vi "check should fail.vi"() -> ()   [LabVIEW 2017]
uses:
  Source/JSON Support for LabVIEW.lvlib
panel:
  out "Array":T1(array[cluster])
  # "Read as"
  # "Parsed As"
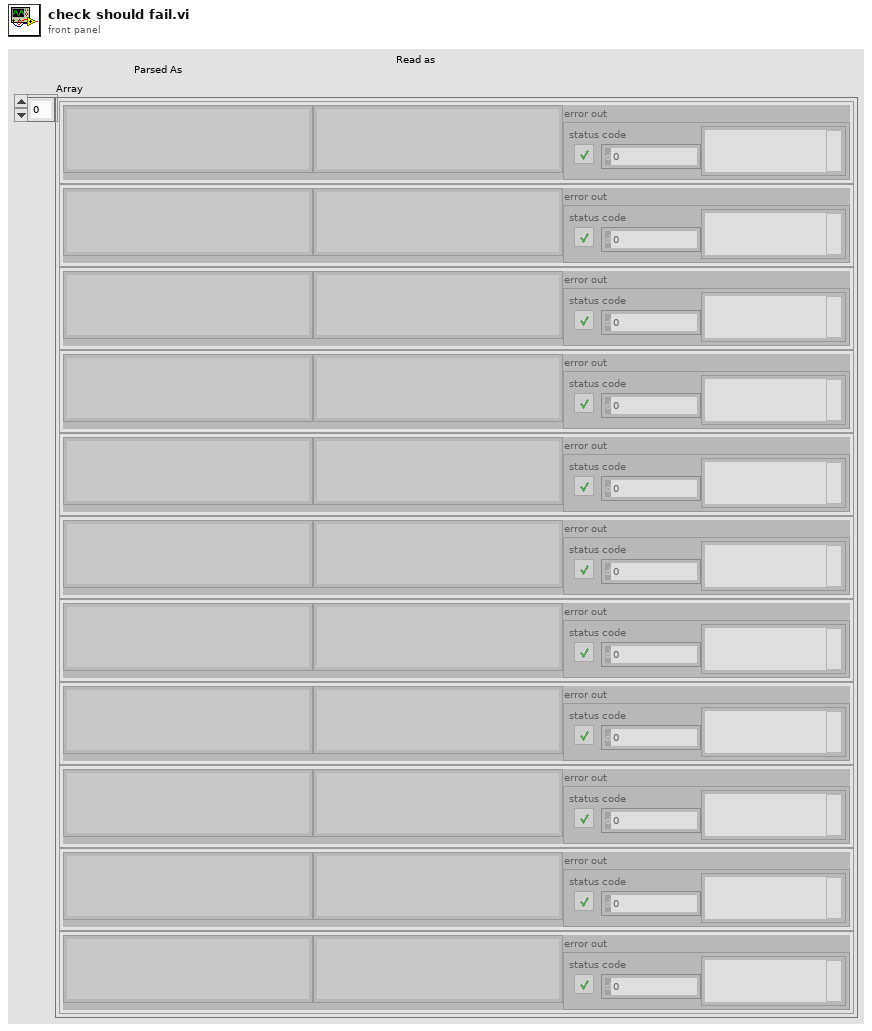
[diagram p1: front panel]
types:
  T1 = cluster{"String":string, string, "error out":errorcluster}[]
  T2 = cluster{"String":string, string, "error out":errorcluster}
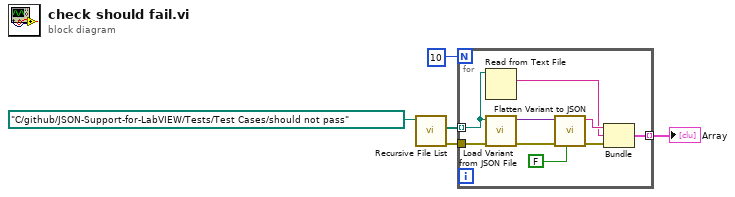
[diagram p0: block diagram]
diagram:
  n1 = call <vilib>:"Recursive File List.vi"("Folder Path"=path "C:/github/JSON-Support-for-LabVIEW/Tests/Test Cases/should not pass" ("Path")) -> ("error out"=w4:errorcluster, "All Files in Dir"=w2:path[])  [unwired: 6 in, 3 out]
  n2 = for {
    N: 10 -> [_]
    tunnel: w2 -> [w11] mode=indexing
    tunnel: w4 -> [w13]
    tunnel: [w8] -> w3 mode=indexing
    n3 = Read from Text File(file (use dialog)=w11) -> (text=w9:string)  [unwired: 3 in, 3 out]
    n4 = call "Load Variant from JSON File.vi"("error in"=w13, "file path"=w11) -> ("error out"=w12:errorcluster, "JSON Value out"=w14:variant)  [unwired: 8 in]
    n5 = call "Flatten Variant to JSON.vi"("pretty print? (F)"=FALSE ("pretty print? (T)"), "error in (no error)"=w12, "JSON Value in"=w14) -> ("error out"=w7:errorcluster, "String"=w10:string)  [unwired: 7 in]
    n6 = Bundle("String"=w10, w9, "error out"=w7) -> (w8:T2)  [unwired: 1 in]
  }
  "Array" <- w3
